vi "5181_Set_RF.vi"(0 "address":string, 1 "center frequency (MHz)":dbl, 2 "modulation (kHz)":i32, 3 "error in (no error)":errorcluster, 4 "amplitude (mV)":i32) -> (5 "address out":string, 6 "error out":errorcluster)   [LabVIEW 2019]
doc: "This device configures the Rohde & Schwarz RF Generator for use. The central frequency, modulation, RF power, and GPIB address are taken from the QCA Global."
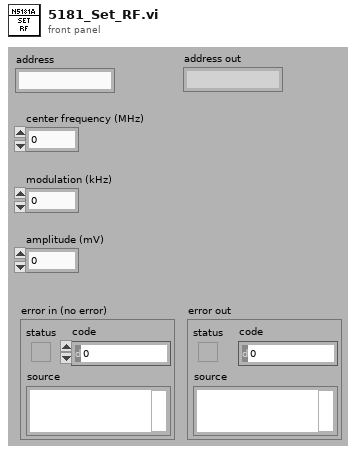
[diagram p1: front panel]
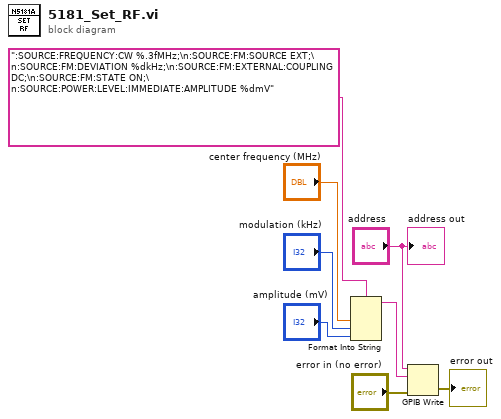
[diagram p0: block diagram]
diagram:
  n1 = Format Into String(format string=":SOURCE:FREQUENCY:CW %.3fMHz;\n:SOURCE:FM:SOURCE EXT;\n:SOURCE:FM:DEVIATION %dkHz;\n:SOURCE:FM:EXTERNAL:COUPLING DC;\n:SOURCE:FM:STATE ON;\n:SOURCE:POWER:LEVEL:IMMEDIATE:AMPLITUDE %dmV", "center frequency (MHz)", "modulation (kHz)", "amplitude (mV)") -> (resulting string=w7:string)  [unwired: 2 in, 1 out]
  n2 = GPIB Write(0:"address", 1:w7, 3:"error in (no error)") -> (6:→"error out":errorcluster)  [unwired: 2 in, 1 out]
  "address out" <- "address"
